vi "Teleop.vi"(10 "Match Info":T1={"Autonomous Elapsed Seconds"=0.0, "TeleOp Elapsed Seconds"=0.0, "Disabled Elapsed Seconds"=0.0, "Visited Autonomous"=FALSE, "Visited TeleOp"=FALSE, "Visited Disabled"=FALSE, "Autonomous Settings"={"Autonomous Style"=enum."Independent", "VI Refnum"=refnum}}, 11 "Call Context":T2) -> ()   [LabVIEW 2014]
doc: "This VI is called for each TeleOp packet received from the DS where the robot is not disabled. It is often used to read from the joysticks and update I/O or to update setpoints for timed control loops. It should complete and return within 20 milliseconds or it may miss DS packets."
uses:
  <vilib>/Rock Robotics/WPI/DriverStation/WPI_DriverStationDerivedRobotMode.ctl
  <vilib>/Rock Robotics/WPI/DriverStation/WPI_DriverStationMatch Info.ctl
  Drivetrain Code/Drivetrain Mode.ctl
  Drivetrain Code/Drivetrain Control.ctl
  Common Code/Change Detect.vi
  Common Code/Change Detect Boolean.vi
  <vilib>/Rock Robotics/WPI/Joystick/WPI_JoystickGetSetRefNum.vi
  Robot Global Data.vi
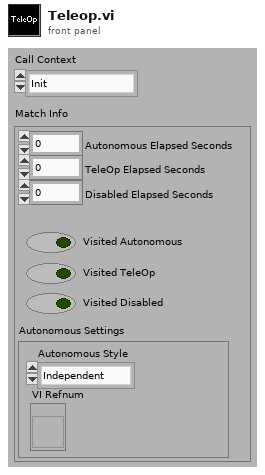
[diagram p1: front panel]
types:
  T1 = typedef "WPI_DriverStationMatch Info.ctl" = cluster{"Autonomous Elapsed Seconds":dbl, "TeleOp Elapsed Seconds":dbl, "Disabled Elapsed Seconds":dbl, "Visited Autonomous":bool, "Visited TeleOp":bool, "Visited Disabled":bool, "Autonomous Settings":cluster{"Autonomous Style":enum16{"Iterative", "Independent"}, "VI Refnum":refnum<vi>}}
  T2 = typedef "WPI_DriverStationDerivedRobotMode.ctl" = enum16{"Init", "Execute", "Stop"}
  T3 = typedef "Drivetrain Mode.ctl" = enum16{"Manual", "Gyro Steer", "Vision Steer", "Drive Distance"}
  T4 = typedef "Drivetrain Control.ctl" = cluster{"Mode":T3, "Steer":dbl, "Y":dbl, "Heading Target":dbl, "Strafe X":dbl, "Y Target":dbl, "Strafe Target":dbl, "X Max Speed":dbl, "X Min Speed":dbl, "Y Max Speed":dbl, "Y Min Speed":dbl}
  T5 = typedef "WPI_JoystickDevRef.ctl" = cluster{"Device":T6}
  T6 = typedef "WPI_JoystickDeviceEnum.ctl" = enum16{"USB 0", "USB 1", "USB 2", "USB 3", "USB 4", "USB 5"}
  T7 = typedef "Button Cluster.ctl" = cluster{"Buttons[0]":bool, "Buttons[1]":bool, "Buttons[2]":bool, "Buttons[3]":bool, "Buttons[4]":bool, "Buttons[5]":bool, "Buttons[6]":bool, "Buttons[7]":bool, "Buttons[8]":bool, "Buttons[9]":bool}
  T8 = typedef "Axes Cluster.ctl" = cluster{"Axes[0]":dbl, "Axes[1]":dbl, "Axes[2]":dbl, "Axes[3]":dbl, "Axes[4]":dbl, "Axes[5]":dbl, "Axes[6]":dbl, "Axes[7]":dbl, "Axes[8]":dbl}
  T9 = typedef "Dashboard Control Data.ctl" = cluster{"Cam Exposure":dbl, "Go to angle":dbl, "Steer PID Gains":cluster{"proportional gain (Kc)":dbl, "integral time (Ti, min)":dbl, "derivative time (Td, min)":dbl}, "Steer PID output Range":cluster{"output high":dbl, "output low":dbl}, "Pressure m \nValue":dbl, "Pressure b \nValue":dbl, "Roller Command Cluster ":T10, "Elevator":T11, "Encoder Control":T13, "Auton Settings":cluster{"Drive Dist Window Size":dbl}, "Drivetrain Settings":T14}
  T10 = typedef "Roller Control.ctl" = cluster{"Intake Speed":dbl, "Turn In Speed":dbl, "Unload Speed":dbl, "Turn Out Speed":dbl, "Ping Align Tolerance":dbl, "Tote Range Threshold":dbl, "Right Pot 0":dbl, "Pot Threshold":dbl, "Left Pot 0":dbl, "Manual 0s?":bool, "Right Pot Scale":dbl, "Left Pot Scale":dbl, "0 wait time":i32, "Zero Pots":bool, "Min Elevator Height":dbl, "Eject Time":dbl, "Eject US Threshold":dbl, "Anti-Twitch Time":u32, "Ping Caring Threshold":dbl, "Pot Diff Threshold":dbl, "Pinch Sustain":u32, "Absorb Give Up Threshold":dbl, "Untip In Threshold":dbl, "Untip Grab Range":dbl, "Ultrasonic Hold Time":u32, "Landscape Absorb Time":u32, "Pot Use Wait Time":u32}
  T11 = typedef "Elevator DB Control.ctl" = cluster{"PID Output Range":cluster{"output high":dbl, "output low":dbl}, "PID gains":cluster{"proportional gain (Kc)":dbl, "integral time (Ti, min)":dbl, "derivative time (Td, min)":dbl}, "Height Tolerance":sgl, " Encoder Constant":dbl, "Safe Mode Max Speed":sgl, "Eject Time":sgl, "Zeroing Speed":sgl, "Presets":T12, "Ping Detect Threshold":sgl, "Trashcan Detect Threshold":sgl, "Zero Filter Time":dbl, "Stabilizer Open Time":dbl, "Zero Creep Speed":dbl, "Max Current":dbl, "Current Trip Time":dbl, "Abort Pitch":dbl}
  T12 = typedef "Elevator Presets.ctl" = cluster{"Pickup 2 w/ Tote":sgl, "Pickup 2 w/ Trashcan":sgl, "Pickup 3 w/ Tote":sgl, "Pickup 3 w/ Trashcan":sgl, "Bottom":sgl, "Pickup 1 w/ Tote":sgl, "Pickup Trashcan":sgl, "Pickup 1 w/ Trashcan":sgl, "Eject":sgl, "Hold Low":sgl, "Step add height":sgl, "Store Trashcan 3":sgl, "Store Trashcan 4":sgl, "Store Trashcan 5":sgl, "6 Tote Max":sgl, "5 Tote Max":sgl, "Untip Lift":dbl, "Drop Stack":dbl, "Pickup 1 Empty":dbl, "Pickup 2 Empty":dbl, "Pickup 3 Empty":dbl, "4 Tote Max":dbl, "HP Load Hold":dbl, "HP Load Drop":dbl}
  T13 = typedef "Encoder Control.ctl" = cluster{"Left Tick Constant":dbl, "Right Tick Constant":dbl, "Center Tick Constant":dbl, "Reset?":bool, "Y Dist":cluster{"PID gains":cluster{"proportional gain (Kc)":dbl, "integral time (Ti, min)":dbl, "derivative time (Td, min)":dbl}}, "X Dist":cluster{"PID gains":cluster{"proportional gain (Kc)":dbl, "integral time (Ti, min)":dbl, "derivative time (Td, min)":dbl}}, "Y Stop Thresh":dbl, "Y Stop Speed":dbl, "X Stop Thresh":dbl, "X Stop Speed":dbl}
  T14 = typedef "Drivetrain Settings.ctl" = cluster{"Gyro Tolerance":dbl, "Strafe Correct max steer":dbl, "Strafe Timer Wait":dbl, "Throttle Ramp (ms)":dbl, "Strafe Ramp (ms)":dbl}
  T15 = typedef "D-Pad.ctl" = cluster{"Top":bool, "Bottom":bool, "None":bool, "Right":bool, "Left":bool}
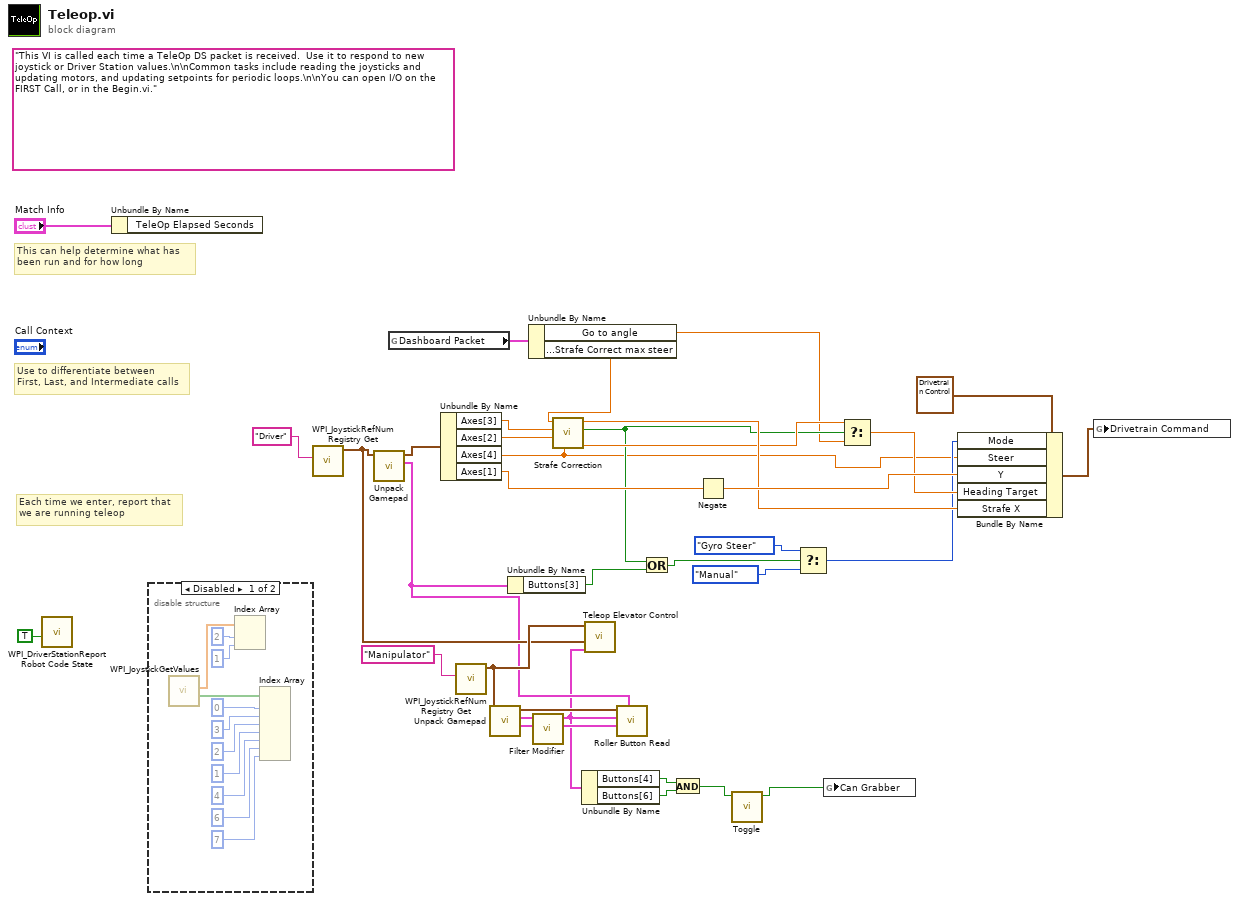
[diagram p0: block diagram]
diagram:
  (unwired) "This VI is called each time a TeleOp DS packet is received.  Use it to respond to new joystick or Driver Station values.\n\nCommon tasks include reading the joysticks and updating motors, and updating setpoints for periodic loops.\n\nYou can open I/O on the FIRST Call, or in the Begin.vi."
  # "Each time we enter, report that\nwe are running teleop"
  # "Use to differentiate between\nFirst, Last, and Intermediate calls"
  # "This can help determine what has\nbeen run and for how long"
  n1 = call <vilib>:"WPI_DriverStationReport Robot Code State.vi"("TeleOp"=TRUE ("Autonomous")) -> ()  [unwired: 10 in, 1 out]
  n2 = Unbundle By Name("Match Info") -> ()  [unwired: 1 out]
  n3 = disable-structure shown="Disabled" {
    frame Disabled {
      n4 = call <vilib>:"WPI_JoystickGetValues.vi"() -> ("Buttons"=w43:bool[], "Axes"=w46:dbl[])  [unwired: 7 in, 3 out]
      n5 = Index Array(array=w46, index #1=2 ("index"), index #2=1 ("index")) -> ()  [unwired: 2 out]
      n6 = Index Array(array=w43, index #1=0 ("index"), index #2=3 ("index"), index #3=2 ("index"), index #4=1 ("index"), index #5=4 ("index"), index #6=6 ("index"), index #7=7 ("index")) -> ()  [unwired: 7 out]
    }
    frame Enabled {
    }
  }
  n7 = call <vilib>:"WPI_JoystickRefNum Registry Get.vi"("refnum name"="Driver") -> ("JoystickDevRef"=w12:T5)  [unwired: 9 in, 1 out]
  n8 = call "Unpack Gamepad.vi"("JoystickDevRef"=w12) -> ("Button Cluster"=w10:T7, "Axes"=w20:T8)  [unwired: 8 in, 1 out]
  n9 = global read "Robot Global Data.vi" "Dashboard Packet"() -> (w5:T9)
  n10 = Unbundle By Name(w20) -> ("Axes[3]"=w23:dbl, "Axes[2]"=w22:dbl, "Axes[4]"=w11:dbl, "Axes[1]"=w21:dbl)
  n11 = call <vilib>:"WPI_JoystickRefNum Registry Get.vi"("refnum name"="Manipulator") -> ("JoystickDevRef"=w30:T5)  [unwired: 9 in, 1 out]
  n12 = call "Unpack Gamepad.vi"("JoystickDevRef"=w30) -> ("D-Pad"=w29:T15, "Button Cluster"=w8:T7, "Axes"=w28:T8)  [unwired: 8 in]
  n13 = Unbundle By Name(w10) -> ("Buttons[3]"=w16:bool)
  n14 = Unbundle By Name(w5) -> ("Go to angle"=w7:dbl, "Drivetrain Settings.Strafe Correct max steer"=w6:dbl)
  n15 = call "Filter Modifier.vi"("Button Cluster 1"=w8) -> ("Button Cluster Out"=w9:T7)  [unwired: 10 in]
  n16 = call "Strafe Correction.vi"("Steer"=w11, "L Trigger"=w22, "R Trigger"=w23, "Max Steer"=w6) -> ("Angle"=w17:dbl, "Gyro Steer"=w14:bool, "Strafe Out"=w24:dbl)  [unwired: 5 in]
  n17 = Unbundle By Name(w9) -> ("Buttons[4]"=w4:bool, "Buttons[6]"=w3:bool)
  n18 = call "Teleop Elevator Control.vi"("Button Cluster"=w9, "Driver Joystick"=w12, "Manipulator Joystick"=w30) -> ()  [unwired: 9 in]
  n19 = call "Roller Button Read.vi"("Driver Button Cluster"=w10, "D-Pad"=w29, "Button Cluster"=w9, "Axes"=w28) -> ()  [unwired: 8 in]
  n20 = Or(x=w14, y=w16) -> (x .or. y?=w13:bool)
  n21 = And(x=w4, y=w3) -> (x .and. y?=w2:bool)
  n22 = Negate(x=w21) -> (-x=w32:dbl)
  n23 = call "Toggle.vi"("In"=w2) -> ("Toggled"=w1:bool)  [unwired: 10 in]
  n24 = Select(t=Drivetrain_Mode."Gyro Steer" ("Mode"), s=w13, f=Drivetrain_Mode."Manual" ("Mode")) -> (s? t:f=w15:T3)
  n25 = global write "Robot Global Data.vi" "Can Grabber"(w1) -> ()
  n26 = Select(t=w17, s=w14, f=w7) -> (s? t:f=w25:dbl)
  n27 = Bundle By Name(cluster=T4 {"Mode"=enum."Gyro Steer", "Steer"=0.0, "Y"=0.0, "Heading Target"=0.0, "Strafe X"=0.0, "Y Target"=0.0, "Strafe Target"=0.0, "X Max Speed"=0.0, "X Min Speed"=0.0, "Y Max Speed"=0.0, "Y Min Speed"=0.0} ("Drivetrain Command"), "Mode"=w15, "Steer"=w11, "Y"=w32, "Heading Target"=w25, "Strafe X"=w24) -> (w33:T4)
  n28 = global write "Robot Global Data.vi" "Drivetrain Command"(w33) -> ()
